vi "Part 1.vi"() -> ()   [LabVIEW 2020]
uses:
  f5607715-37ea-46d8-9f6d-9d0be51d8b73.vi
panel:
  out "x+y":dbl
  in  "x":dbl
  in  "y":dbl
  out "size(s)":i32
  out "Answer":T1(array[cluster])
  in  "Sum":i32
  out "Array":i32[](array[numeric])
  in  "Numbers":i32
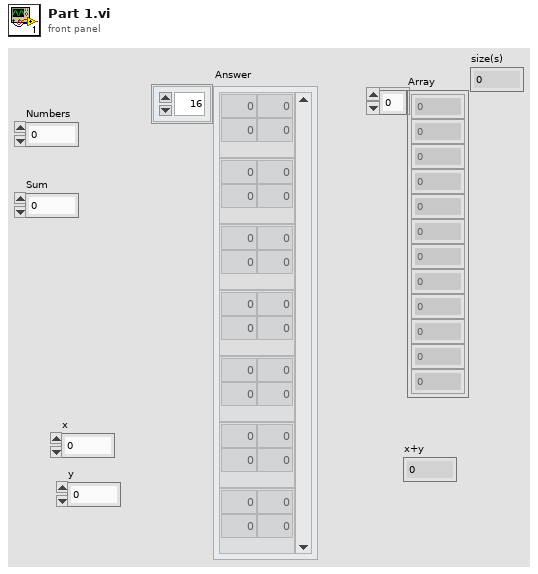
[diagram p1: front panel]
types:
  T1 = cluster{"Number 1":dbl, "Number 2":dbl, "Number 3":dbl, "Number 4":dbl}[]
  T2 = cluster{"[0]":i32, "[1]":i32, "[2]":i32, "[3]":i32}
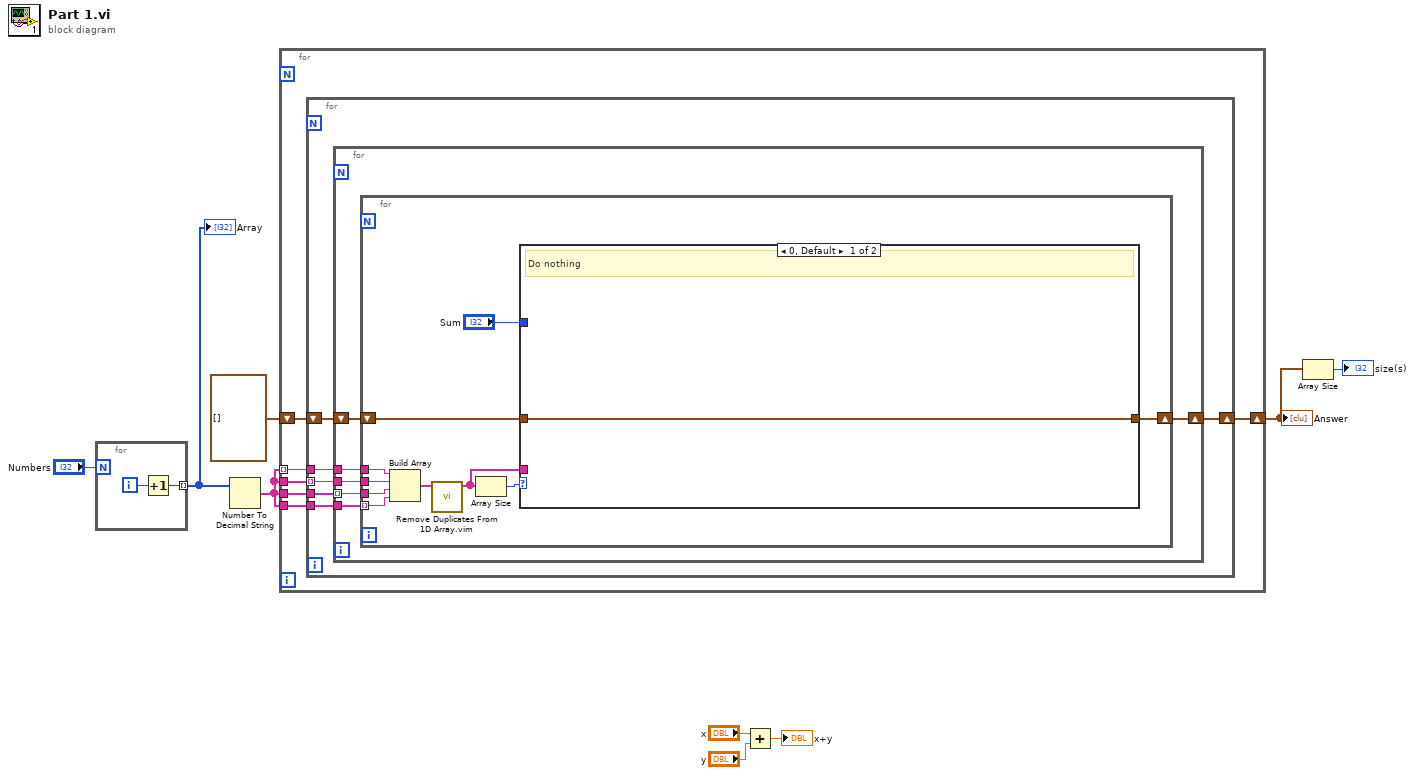
[diagram p0: block diagram]
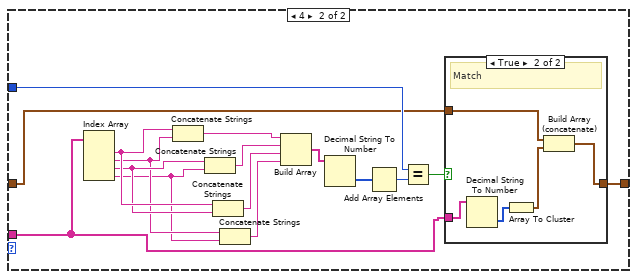
[diagram p2: hidden frame]
diagram:
  n1 = for {
    N: "Numbers" -> [_]
    tunnel: [w10] -> w8 mode=indexing
    i -> [w11]
    n2 = Increment(x=w11) -> (x+1=w10:i32)
  }
  "Array" <- w8
  n3 = Number To Decimal String(number=w8) -> (decimal integer string=w7:string[])  [unwired: 1 in]
  n4 = for {
    tunnel: w7 -> [w17] mode=indexing
    tunnel: w7 -> [w16]
    tunnel: w7 -> [w15]
    tunnel: w7 -> [w14]
    shift-right: [w12] -> w5
    shift-left: T1 [] ("Answer") -> [w13]
    n5 = for {
      tunnel: w17 -> [w23]
      tunnel: w16 -> [w22] mode=indexing
      tunnel: w15 -> [w21]
      tunnel: w14 -> [w20]
      shift-right: [w18] -> w12
      shift-left: w13 -> [w19]
      n6 = for {
        tunnel: w23 -> [w29]
        tunnel: w22 -> [w28]
        tunnel: w21 -> [w27] mode=indexing
        tunnel: w20 -> [w26]
        shift-right: [w24] -> w18
        shift-left: w19 -> [w25]
        n7 = for {
          tunnel: w29 -> [w39]
          tunnel: w28 -> [w38]
          tunnel: w27 -> [w37]
          tunnel: w26 -> [w36] mode=indexing
          shift-right: [w32] -> w24
          shift-left: w25 -> [w31]
          n8 = Build Array(w39, w38, w37, w36) -> (w35:string[])
          n9 = call "Remove Duplicates From 1D Array.vim"("array"=w35) -> ("array with duplicates removed"=w33:string[])  [unwired: 10 in]
          n10 = Array Size(array=w33) -> (size(s)=w34:i32)
          n11 = case shown="0, Default" w34 {
            tunnel: w33 -> [_ w41]
            tunnel: [w40 w43] -> w32
            tunnel: w31 -> [w40 w42]
            tunnel: "Sum" -> [_ w45]
            frame 0, Default {
              # "Do nothing"
            }
            frame 4 {
              n12 = Index Array(array=w41) -> (element #1=w56:string, element #2=w54:string, element #3=w55:string, element #4=w53:string)  [unwired: 4 in]
              n13 = Concatenate Strings(w56, w54) -> (w52:string)
              n14 = Concatenate Strings(w55, w53) -> (w51:string)
              n15 = Concatenate Strings(w56, w55) -> (w50:string)
              n16 = Concatenate Strings(w54, w53) -> (w49:string)
              n17 = Build Array(w52, w51, w50, w49) -> (w48:string[])
              n18 = Decimal String To Number(string=w48) -> (number=w47:i32[])  [unwired: 2 in, 1 out]
              n19 = Add Array Elements(numeric array=w47) -> (sum=w46:i32)
              n20 = Equal?(x=w45, y=w46) -> (x = y?=w44:bool)
              n21 = case shown="True" w44 {
                tunnel: [w57 w58] -> w43
                tunnel: w42 -> [w57 w60]
                tunnel: w41 -> [_ w62]
                frame False {
                }
                frame True {
                  # "Match"
                  n22 = Decimal String To Number(string=w62) -> (number=w61:i32[])  [unwired: 2 in, 1 out]
                  n23 = Array To Cluster(array=w61) -> (cluster=w59:T2)
                  n24 = Build Array (concatenate)(w60, w59) -> (w58:T1)
                }
              }
            }
          }
        }
      }
    }
  }
  "Answer" <- w5
  n25 = Add(x="x", y="y") -> (x+y=→"x+y":dbl)
  n26 = Array Size(array=w5) -> (size(s)=→"size(s)":i32)
